vi "R4Initialize.vi"(8 "error in (no error)":errorcluster) -> (0 "error out":errorcluster)   [LabVIEW 2016]
uses:
  Controls/pH_SetParams Standard.ctl
  R4Controls/R4SBR_SetParams.ctl
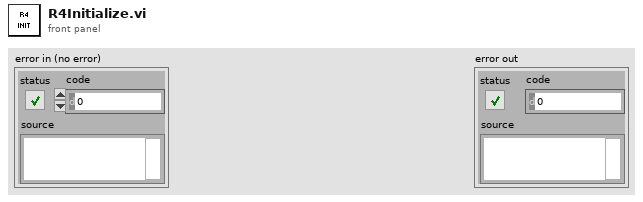
[diagram p1: front panel]
types:
  T1 = typedef "R4SBR_SetParams.ctl" = cluster{"Phase":string, "Time, min":dbl, "SBR_Manual (Standard)":cluster{"Media Pump":bool, "Water Pump":bool, "Gas Pump":bool, "Effluent Pump":bool, "Release Pump":bool}}[]
  T2 = cluster{"Media Pump":bool, "Water Pump":bool, "Effluent Pump":bool, "Release Valve":bool, "Gas Pump":bool}
  T3 = cluster{"Set Point, mg/L":dbl, "Tolerance, mg/L":dbl, "N2 Valve Gain":dbl, "Air Valve Gain":dbl}
  T4 = typedef "pH_SetParams Standard.ctl" = cluster{"Set Point":dbl, "Tolerance":dbl, "Pump Time On, secs":dbl}
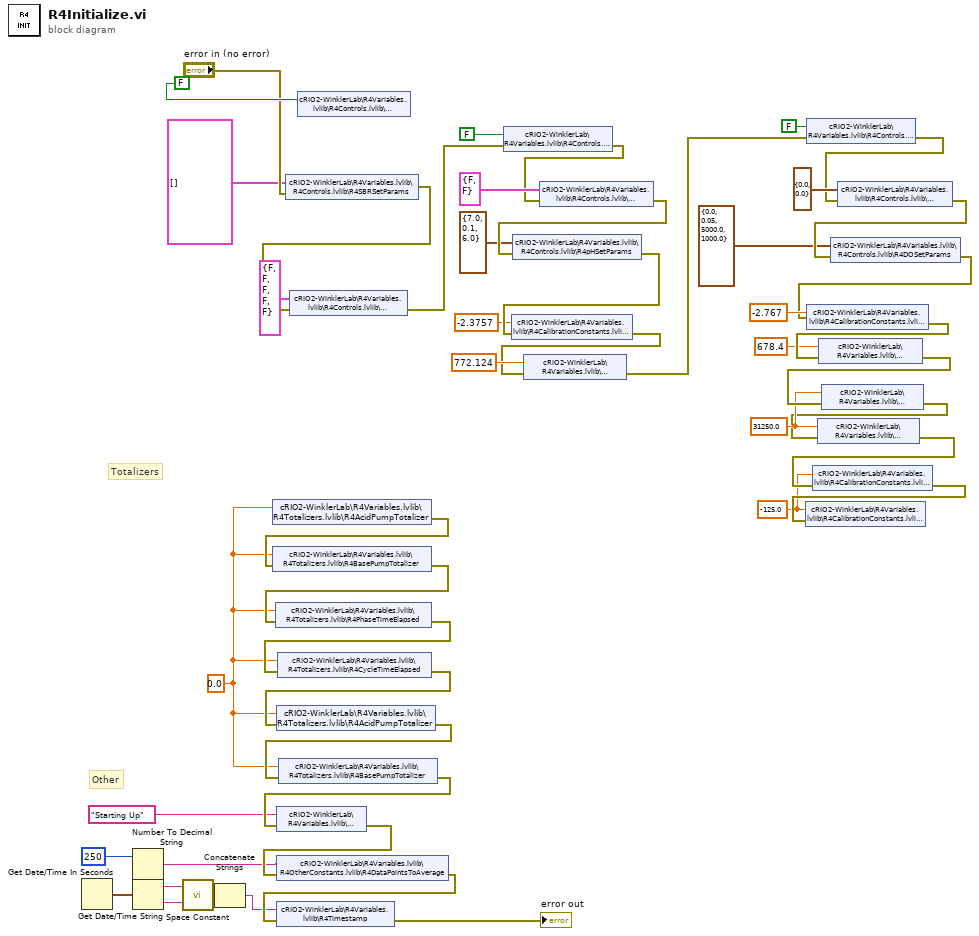
[diagram p0: block diagram]
diagram:
  w10 = 0.0 ("R1PhaseTimeElapsed")
  w20 = 31250.0 ("R1AirSlope")
  w16 = -125.0 ("R1N2Intercept")
  # "Totalizers"
  # "Other"
  n1 = Get Date/Time In Seconds() -> (seconds since 1Jan1904=w48:timestamp)
  n2 = Number To Decimal String(number=250 ("R1DataPointsToAverage")) -> (decimal integer string=w4:string)  [unwired: 1 in]
  n3 = Get Date/Time String(seconds (now)=w48) -> (date string=w45:string, time string=w47:string)  [unwired: 2 in]
  n4 = call <vilib>:"Space Constant.vi"() -> ("String"=w46:string)
  n5 = Concatenate Strings(w45, w46, w47) -> (w3:string)
  n6 = shared-variable "cRIO2-WinklerLab\\R4Variables.lvlib\\R4Totalizers.lvlib\\R4AcidPumpTotalizer"(w10) -> (error out=w15:errorcluster)  [unwired: 1 in]
  n7 = shared-variable "cRIO2-WinklerLab\\R4Variables.lvlib\\R4Totalizers.lvlib\\R4BasePumpTotalizer"(w10, error in=w15) -> (error out=w14:errorcluster)
  n8 = shared-variable "cRIO2-WinklerLab\\R4Variables.lvlib\\R4Totalizers.lvlib\\R4PhaseTimeElapsed"(w10, error in=w14) -> (error out=w13:errorcluster)
  n9 = shared-variable "cRIO2-WinklerLab\\R4Variables.lvlib\\R4Totalizers.lvlib\\R4CycleTimeElapsed"(w10, error in=w13) -> (error out=w12:errorcluster)
  n10 = shared-variable "cRIO2-WinklerLab\\R4Variables.lvlib\\R4Totalizers.lvlib\\R4AcidPumpTotalizer"(w10, error in=w12) -> (error out=w11:errorcluster)
  n11 = shared-variable "cRIO2-WinklerLab\\R4Variables.lvlib\\R4Totalizers.lvlib\\R4BasePumpTotalizer"(w10, error in=w11) -> (error out=w9:errorcluster)
  n12 = shared-variable "cRIO2-WinklerLab\\R4Variables.lvlib\\R4Status"("Starting Up" ("R1Status"), error in=w9) -> (error out=w8:errorcluster)
  n13 = shared-variable "cRIO2-WinklerLab\\R4Variables.lvlib\\R4OtherConstants.lvlib\\R4DataPointsToAverage"(w4, error in=w8) -> (error out=w6:errorcluster)
  n14 = shared-variable "cRIO2-WinklerLab\\R4Variables.lvlib\\R4Timestamp"(w3, error in=w6) -> (error out=→"error out":errorcluster)
  n15 = shared-variable "cRIO2-WinklerLab\\R4Variables.lvlib\\R4Controls.lvlib\\R4SBRSetParams"(T1 [] ("R4SBR_SetParams"), error in="error in (no error)") -> (error out=w42:errorcluster)
  n16 = shared-variable "cRIO2-WinklerLab\\R4Variables.lvlib\\R4Controls.lvlib\\R4SBRManual"(T2 {"Media Pump"=FALSE, "Water Pump"=FALSE, "Effluent Pump"=FALSE, "Release Valve"=FALSE, "Gas Pump"=FALSE} ("R4SBRManual"), error in=w42) -> (error out=w40:errorcluster)
  n17 = shared-variable "cRIO2-WinklerLab\\R4Variables.lvlib\\R4Controls.lvlib\\R4SBRSwitch"(FALSE ("R1SBRSwitch")) -> ()  [unwired: 1 in, 1 out]
  n18 = shared-variable "cRIO2-WinklerLab\\R4Variables.lvlib\\R4Controls.lvlib\\R4pHSwitch"(FALSE ("R1pHSwitch"), error in=w40) -> (error out=w38:errorcluster)
  n19 = shared-variable "cRIO2-WinklerLab\\R4Variables.lvlib\\R4Controls.lvlib\\R4pHManual"(cluster{"Acid Pump":bool, "Base Pump":bool} {"Acid Pump"=FALSE, "Base Pump"=FALSE} ("R1pHManual"), error in=w38) -> (error out=w37:errorcluster)
  n20 = shared-variable "cRIO2-WinklerLab\\R4Variables.lvlib\\R4Controls.lvlib\\R4pHSetParams"(T4 {"Set Point"=7.0, "Tolerance"=0.1, "Pump Time On, secs"=6.0} ("R1pHSetParams"), error in=w37) -> (error out=w35:errorcluster)
  n21 = shared-variable "cRIO2-WinklerLab\\R4Variables.lvlib\\R4CalibrationConstants.lvlib\\R4pHIntercept"(-2.3757 ("R12pHInt"), error in=w35) -> (error out=w32:errorcluster)
  n22 = shared-variable "cRIO2-WinklerLab\\R4Variables.lvlib\\R4CalibrationConstants.lvlib\\R4pHSlope"(772.124 ("R1pHSlope"), error in=w32) -> (error out=w30:errorcluster)
  n23 = shared-variable "cRIO2-WinklerLab\\R4Variables.lvlib\\R4Controls.lvlib\\R4pHSwitch"(FALSE ("R1pHSwitch"), error in=w30) -> (error out=w28:errorcluster)
  n24 = shared-variable "cRIO2-WinklerLab\\R4Variables.lvlib\\R4Controls.lvlib\\R4DOManual"(cluster{"Air MFC":dbl, "N2 MFC":dbl} {"Air MFC"=0.0, "N2 MFC"=0.0} ("R1DOManual"), error in=w28) -> (error out=w27:errorcluster)
  n25 = shared-variable "cRIO2-WinklerLab\\R4Variables.lvlib\\R4Controls.lvlib\\R4DOSetParams"(T3 {"Set Point, mg/L"=0.0, "Tolerance, mg/L"=0.05, "N2 Valve Gain"=5000.0, "Air Valve Gain"=1000.0} ("R1DOSetParams"), error in=w27) -> (error out=w24:errorcluster)
  n26 = shared-variable "cRIO2-WinklerLab\\R4Variables.lvlib\\R4CalibrationConstants.lvlib\\R4DOIntercept"(-2.767 ("R1DOInt"), error in=w24) -> (error out=w23:errorcluster)
  n27 = shared-variable "cRIO2-WinklerLab\\R4Variables.lvlib\\R4CalibrationConstants.lvlib\\R4DOSlope"(678.4 ("R1DOSlope"), error in=w23) -> (error out=w21:errorcluster)
  n28 = shared-variable "cRIO2-WinklerLab\\R4Variables.lvlib\\R4CalibrationConstants.lvlib\\R4N2Slope"(w20, error in=w21) -> (error out=w19:errorcluster)
  n29 = shared-variable "cRIO2-WinklerLab\\R4Variables.lvlib\\R4CalibrationConstants.lvlib\\R4AirSlope"(w20, error in=w19) -> (error out=w18:errorcluster)
  n30 = shared-variable "cRIO2-WinklerLab\\R4Variables.lvlib\\R4CalibrationConstants.lvlib\\R4AirIntercept"(w16, error in=w18) -> (error out=w17:errorcluster)
  n31 = shared-variable "cRIO2-WinklerLab\\R4Variables.lvlib\\R4CalibrationConstants.lvlib\\R4N2Intercept"(w16, error in=w17) -> ()  [unwired: 1 out]
